vi "Proxy Server Info.vi"(8 "error in (no error)":errorcluster, 9 "Get/Set":enum16{"Get", "Set"}(ring), 11 "Proxy Server Info":T1) -> (0 "error out":errorcluster, 3 "Proxy Server Info 2":T1)   [LabVIEW 2020, in "WebServiceImporter.lvlib" / "ProxyDll Generator.lvlib"]
uses:
  <vilib>/Platform/WebService/ProxyDll Generator/ProxyDll Generator.lvlib
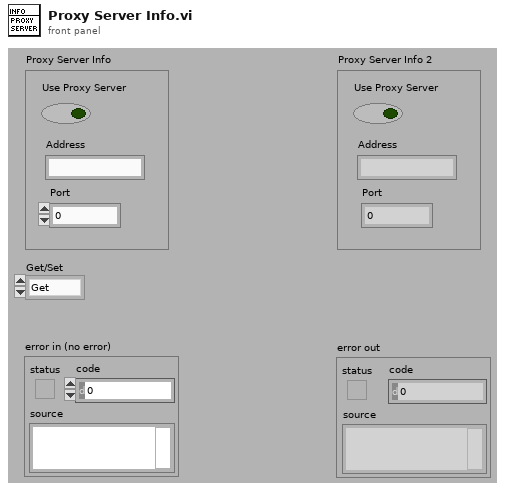
[diagram p1: front panel]
types:
  T1 = cluster{"Use Proxy Server":bool, "Address":string, "Port":u32}
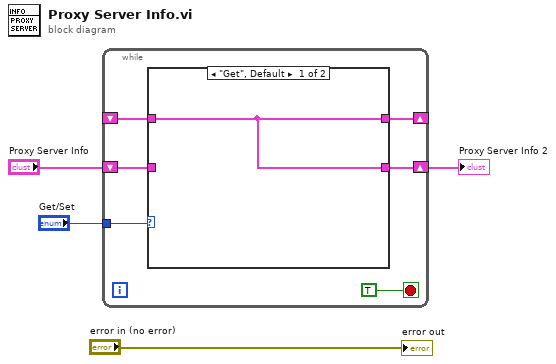
[diagram p0: block diagram]
diagram:
  n1 = while {
    tunnel: "Get/Set" -> [w9]
    shift-right: [w7] -> w1
    shift-left: "Proxy Server Info" -> [w8]
    shift-right: [w6] -> _
    shift-left: _ -> [w5]
    stop <- TRUE stop-if-true
    n2 = case shown="\"Get\", Default" w9 {
      tunnel: w8 -> [_ w12]
      tunnel: [w11 w12] -> w7
      tunnel: [w11 w12] -> w6
      tunnel: w5 -> [w11 _]
      frame "Get", Default {
      }
      frame "Set" {
      }
    }
  }
  "Proxy Server Info 2" <- w1
  "error out" <- "error in (no error)"
